vi "SubInitializeDlg.vi"(8 "error in (no error)":errorcluster, 9 "modes of operations":i8(ring)=1 items=["Profile Position Mode"=1, "Profile Velocity Mode"=3, "Homing Mode"=6, "Interpolated Position Mode"=7, "Position Mode"=-1, "Velocity Mode"=-2, "Current Mode"=-3, "Master Encoder Mode"=-5, "Step Direction Mode"=-6], 10 "nodeId":u16=2, 11 "axis in":cluster{"keyHandle":u32, "nodeId":u16}={"keyHandle"=0, "nodeId"=1}) -> (0 "error out":errorcluster, 3 "axis out":cluster{"keyHandle":u32, "nodeId":u16}={"keyHandle"=0, "nodeId"=1})   [LabVIEW 2019, in "maxonEPOS.lvlib"]
doc: "<B>InitializeDlg</B> registers available interfaces (CAN, USB and RS232) with which the EPOS can be operated and opens the selected interface for communication.\nThe function sets a new operational mode and clears all errors from a connected node."
uses:
  Examples/maxonEPOS.lvlib
panel:
  in  "baudrate":u32=1000000
  # "(c) 2007 - 2017 maxon motor ag.  ALL RIGHTS RESERVED."
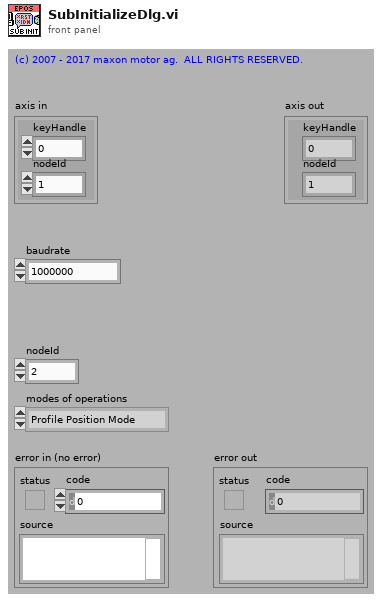
[diagram p1: front panel]
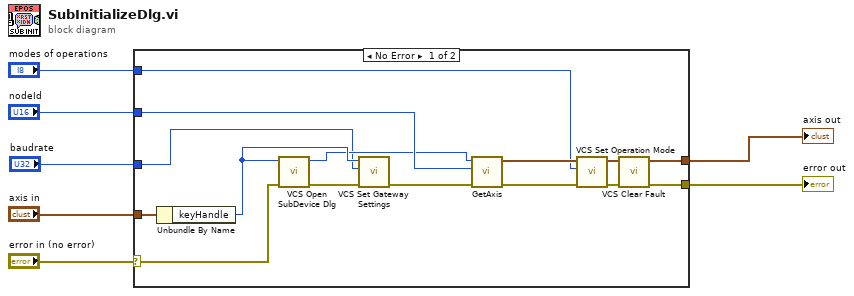
[diagram p0: block diagram]
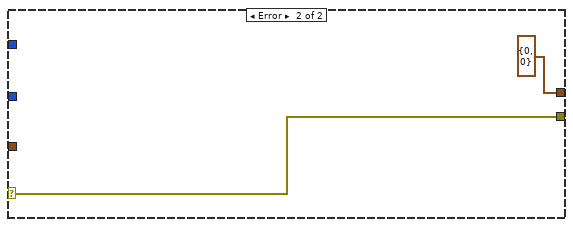
[diagram p2: hidden frame]
diagram:
  n1 = case shown="No Error" "error in (no error)" {
    selector: "error in (no error)" -> [w11 w24]
    tunnel: [w20 w24] -> w6
    tunnel: [w19 cluster{"keyHandle":u32, "nodeId":u16} {"keyHandle"=0, "nodeId"=0} ("axis out")] -> w5
    tunnel: "nodeId" -> [w16 _]
    tunnel: "modes of operations" -> [w15 _]
    tunnel: "axis in" -> [w14 _]
    tunnel: "baudrate" -> [w8 _]
    frame No Error {
      n2 = Unbundle By Name(w14) -> ("keyHandle"=w13:u32)
      n3 = call "VCS Open SubDevice Dlg.vi"("error in (no error)"=w11, "deviceHandle"=w13) -> ("error out"=w10:errorcluster, "keyHandle"=w12:u32)  [unwired: 8 in]
      n4 = call "VCS Set Gateway Settings.vi"("error in (no error)"=w10, "Baudrate"=w8, "keyHandle in"=w13) -> ("error out"=w9:errorcluster)  [unwired: 7 in, 1 out]
      n5 = call "GetAxis.vi"("error in (no error)"=w9, "nodeId"=w16, "keyHandle in"=w12) -> ("error out"=w22:errorcluster, "axis out"=w17:cluster{"keyHandle":u32, "nodeId":u16})  [unwired: 7 in]
      n6 = call "VCS Set Operation Mode.vi"("error in (no error)"=w22, "modes of operations"=w15, "axis in"=w17) -> ("error out"=w21:errorcluster, "axis out"=w18:cluster{"keyHandle":u32, "nodeId":u16})  [unwired: 7 in]
      n7 = call "VCS Clear Fault.vi"("error in (no error)"=w21, "axis in"=w18) -> ("error out"=w20:errorcluster, "axis out"=w19:cluster{"keyHandle":u32, "nodeId":u16})  [unwired: 8 in]
    }
    frame Error {
    }
  }
  "error out" <- w6
  "axis out" <- w5
